vi "Read Log (popup).vi"(8 "error in (no error)":errorcluster, 11 "file path (use dialog)":path) -> (0 "error out":errorcluster)   [LabVIEW 2012]
panel:
  out "Table":string[][](table)
  in  "Save":bool
  in  "Exit":bool
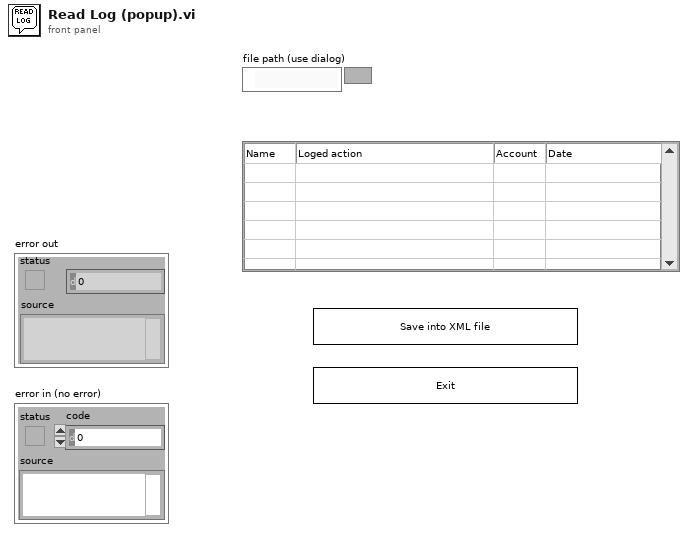
[diagram p1: front panel]
types:
  T1 = enum16{"open", "replace", "create", "open or create", "replace or create", "replace or create with confirmation"}
  T2 = typedef "Log_User_Data.ctl" = cluster{"User":string, "Action":string, "Account type":T3, "Login Time ":timestamp}
  T3 = typedef "User Accounts.ctl" = enum16{"None", "User", "Admin"}
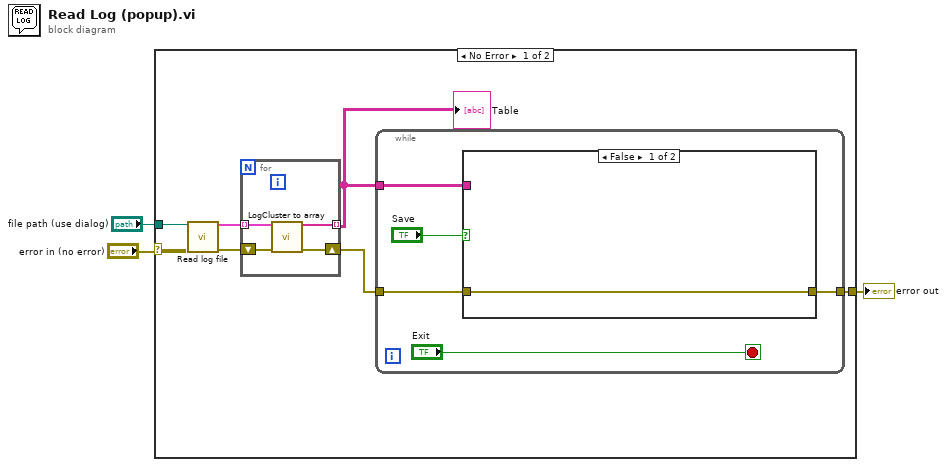
[diagram p0: block diagram]
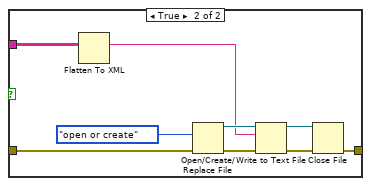
[diagram p2: hidden frame]
diagram:
  n1 = case shown="No Error" "error in (no error)" {
    selector: "error in (no error)" -> [w7 w30]
    tunnel: [w10 w30] -> w3
    tunnel: "file path (use dialog)" -> [w8 _]
    frame No Error {
      n2 = call "Read log file.vi"("file path (use dialog)"=w8, "error in"=w7) -> ("Array"=w9:T2[], "error out"=w6:errorcluster)  [unwired: 12 in]
      n3 = for {
        tunnel: [w14] -> w4 mode=indexing
        tunnel: w9 -> [w11] mode=indexing
        shift-right: [w13] -> w5
        shift-left: w6 -> [w12]
        n4 = call "LogCluster to array.vi"("Log Cluster"=w11, "error in (no error)"=w12) -> ("Log array"=w14:string[], "error out"=w13:errorcluster)  [unwired: 12 in]
      }
      "Table" <- w4
      n5 = while {
        tunnel: w4 -> [w17]
        tunnel: [w16] -> w10
        tunnel: w5 -> [w15]
        stop <- "Exit" stop-if-true
        n6 = case shown="False" "Save" {
          tunnel: w17 -> [_ w23]
          tunnel: [w20 w22] -> w16
          tunnel: w15 -> [w20 w21]
          frame False {
          }
          frame True {
            n7 = Flatten To XML(anything=w23) -> (xml string=w24:string)
            n8 = Open/Create/Replace File(error in=w21, operation (0:open)=T1."open or create") -> (refnum out=w28:refnum<file>, error out=w27:errorcluster)  [unwired: 4 in, 1 out]
            n9 = Write to Text File(file (use dialog)=w28, text=w24, error in=w27) -> (refnum out=w26:refnum<file>, error out=w25:errorcluster)  [unwired: 1 in, 1 out]
            n10 = Close File(refnum=w26, error in=w25) -> (error out=w22:errorcluster)  [unwired: 1 out]
          }
        }
      }
    }
    frame Error {
    }
  }
  "error out" <- w3
